vi "Single Calculate Mask Test Gate Time Query.vi"(8 "error in":errorcluster, 10 "Calculation Channel":i32(ring) items=["Calc Channel 1", "Calc Channel 2", "Calc Channel 3", "Calc Channel 4"], 11 "Instrument Handle In":i32) -> (0 "error out":errorcluster, 1 "Stop":dbl, 2 "Start":dbl, 3 "Instrument Handle Out":i32)   [LabVIEW 8.6, in "ZTScopeM.lvlib"]
doc: "Returns the mask gate limits for the selected channel in time."
uses:
  ZTScopeM.lvlib
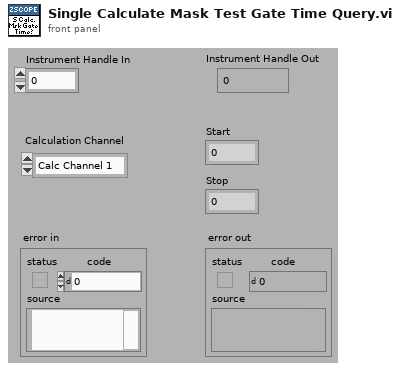
[diagram p1: front panel]
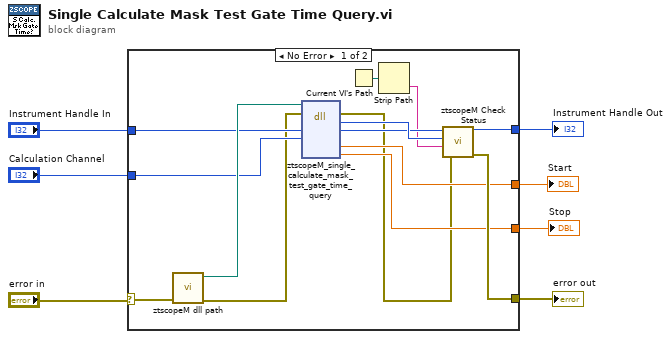
[diagram p0: block diagram]
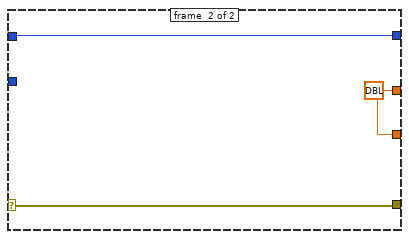
[diagram p2: hidden frame]
diagram:
  n1 = case shown="No Error" "error in" {
    selector: "error in" -> [w13 w24]
    tunnel: [w16 w24] -> w6
    tunnel: [w17 w22] -> w5
    tunnel: [w15 w23] -> w4
    tunnel: [w14 w23] -> w3
    tunnel: "Instrument Handle In" -> [w11 w22]
    tunnel: "Calculation Channel" -> [w10 _]
    frame #0 {
      n2 = call "ztscopeM dll path.vi"("error in (no error)"=w13) -> ("error out"=w9:errorcluster, "<instrument>.dll path"=w12:path)  [unwired: 9 in]
      n3 = dll-call lib="C:/Program Files (x86)/National Instruments/LabVIEW 2013/instr.lib/ztscopem/ztscopeM.dll" fn="ztscopeM_single_calculate_mask_test_gate_time_query"(path in=w12, error in=w9, "instrumentHandle"=w11, "calculationChannel"=w10) -> (error out=w8:errorcluster, w21:i32, "instrumentHandle"=w20:i32, "start"=w15:dbl, "stop"=w14:dbl)  [unwired: 2 in, 3 out]
      n4 = Current VI's Path() -> (path=w19:path)
      n5 = Strip Path(path=w19) -> (name=w18:string)  [unwired: 1 out]
      n6 = call "ztscopeM Check Status.vi"("error in"=w8, "name of VI"=w18, "status (return code)"=w21, "instrument handle in"=w20) -> ("error out"=w16:errorcluster, "instrument handle out"=w17:i32)  [unwired: 2 out]
    }
    frame #1 {
      w23 = dbl ? ("start")
    }
  }
  "Instrument Handle Out" <- w5
  "error out" <- w6
  "Start" <- w4
  "Stop" <- w3
